vi "值已改变(Boolean).vi"(1 "初始化":bool, 3 "输入数据":bool) -> (0 "已更改":bool)   [LabVIEW 2012]
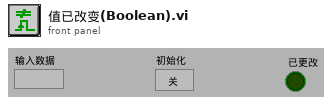
[diagram p1: front panel]
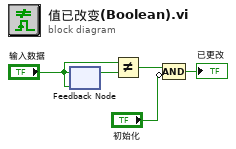
[diagram p0: block diagram]
diagram:
  n1 = feedback-in #1("输入数据") -> ()
  n2 = feedback #1("输入数据") -> (w4:bool)
  n3 = Not Equal?(x="输入数据", y=w4) -> (x != y?=w3:bool)
  n4 = Compound Arithmetic op=AND(w3, invert "初始化") -> (→"已更改":bool)
